vi "Get Current Draw.vi"(8 "error in (no error)":errorcluster, 11 "Simulated PSU in":refnum<class "Simulated PSU.lvclass">) -> (0 "error out":errorcluster, 2 "Current Draw (Amps)":dbl, 3 "Simulated PSU out":refnum<class "Simulated PSU.lvclass">)   [LabVIEW 2020, in "Simulated PSU.lvlib" / "Simulated PSU.lvclass"]
uses:
  Simulated PSU.lvclass
  Simulated PSU.lvclass/Simulated PSU.ctl
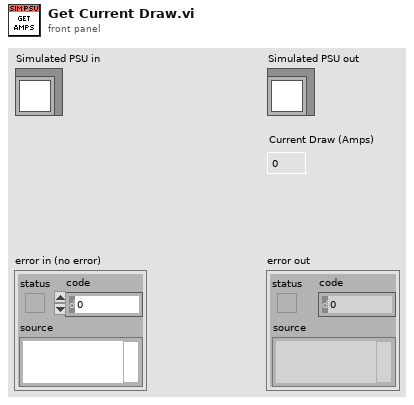
[diagram p1: front panel]
types:
  T1 = typedef "Simulated PSU.lvlib/Simulated PSU.lvclass/Ref Data.ctl" = cluster{"Enabled":bool, "Voltage":dbl, "Noise Level":dbl, "Resistance":dbl}
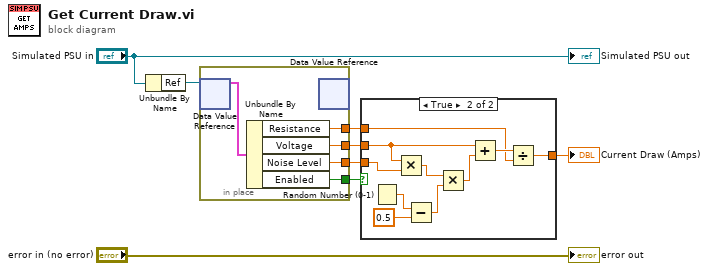
[diagram p0: block diagram]
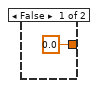
[diagram p2: hidden frame]
diagram:
  n1 = Unbundle By Name("Simulated PSU in") -> ("Ref"=w7:refnum<data-value>)
  n2 = in-place {
    in-place-border: [w12] -> w2
    in-place-border: [w11] -> w3
    in-place-border: [w10] -> w4
    in-place-border: [w9] -> w5
    n3 = in-place-dvr #1(w7) -> (w13:T1)  [unwired: 1 out]
    n4 = Unbundle By Name(w13) -> ("Resistance"=w12:dbl, "Voltage"=w11:dbl, "Noise Level"=w10:dbl, "Enabled"=w9:bool)
    n5 = in-place-dvr #1() -> ()  [unwired: 1 in, 2 out]
  }
  n6 = case shown="True" w5 {
    tunnel: w4 -> [_ w24]
    tunnel: w3 -> [_ w19]
    tunnel: w2 -> [_ w16]
    tunnel: [0.0 w15] -> w1
    frame False {
    }
    frame True {
      n7 = Random Number (0-1)() -> (number: 0 to 1=w22:dbl)
      n8 = Multiply(x=w19, y=w24) -> (x*y=w23:dbl)
      n9 = Subtract(x=w22, y=0.5) -> (x-y=w20:dbl)
      n10 = Multiply(x=w23, y=w20) -> (x*y=w18:dbl)
      n11 = Add(x=w19, y=w18) -> (x+y=w17:dbl)
      n12 = Divide(x=w17, y=w16) -> (x/y=w15:dbl)
    }
  }
  "Current Draw (Amps)" <- w1
  "error out" <- "error in (no error)"
  "Simulated PSU out" <- "Simulated PSU in"
